vi "De-Normalize Rectangle.vi"(10 "X Resolution":i32, 11 "Right":dbl) -> (3 "Pixels":dbl)   [LabVIEW 2015]
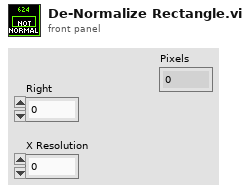
[diagram p1: front panel]
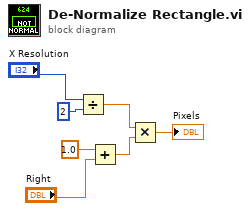
[diagram p0: block diagram]
diagram:
  n1 = Divide(x="X Resolution", y=2) -> (x/y=w6:dbl)
  n2 = Add(x=1.0, y="Right") -> (x+y=w7:dbl)
  n3 = Multiply(x=w6, y=w7) -> (x*y=→"Pixels":dbl)
